vi "Set speed at 70.vi"(8 "error in (no error)":errorcluster, 9 "Axis (1..4)":u16(ring)=1 items=["X"=1, "Y"=2, "Z"=3, "Rotary"=4], 10 "Speed at 70%, counts/s":i32=2000, 11 "VISA resource name":refnum<visa-resource-name>="COM11") -> (0 "error out":errorcluster={"status"=FALSE, "code"=1073676294, "source"="VISA Read in VXM Com.vi->Set speed at 70.vi"}, 3 "VISA resource out":refnum<visa-resource-name>="COM11")   [LabVIEW 2017]
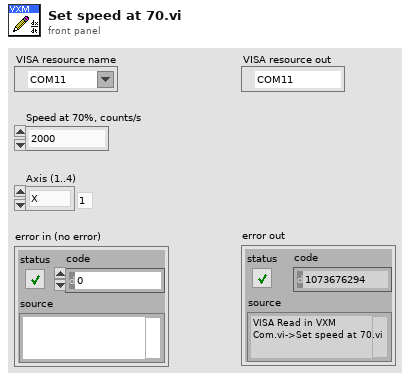
[diagram p1: front panel]
types:
  T1 = enum16{"Cmd-Response", "Write Only", "Read Only"}
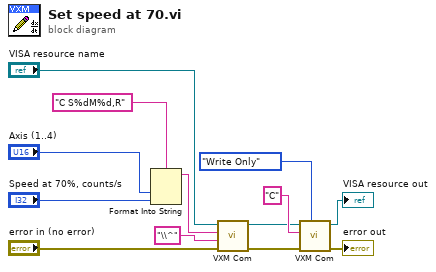
[diagram p0: block diagram]
diagram:
  n1 = Format Into String(format string="C S%dM%d,R" ("Command"), "Axis (1..4)", "Speed at 70%, counts/s") -> (resulting string=w11:string)  [unwired: 2 in, 1 out]
  n2 = call "VXM Com.vi"("error in (no error)"="error in (no error)", "Termination String ('/' codes)"="\\^", "Write Buffer ('/' codes)"=w11, "VISA resource name"="VISA resource name") -> ("error out"=w2:errorcluster, "VISA resource out"=w1:refnum<visa-resource-name>)  [unwired: 5 in, 1 out]
  n3 = call "VXM Com.vi"("Operation"=T1."Write Only", "error in (no error)"=w2, "Write Buffer ('/' codes)"="C" ("Write Buffer"), "VISA resource name"=w1) -> ("error out"=→"error out":errorcluster, "VISA resource out"=→"VISA resource out":refnum<visa-resource-name>)  [unwired: 5 in, 1 out]
